vi "read_data_from_fieldpoint.vi"(8 "error in (no error)":errorcluster, 11 "fieldpoint_rw in":refnum<class "fieldpoint_rw.lvclass">) -> (0 "error out":errorcluster, 3 "fieldpoint_rw out":refnum<class "fieldpoint_rw.lvclass">)   [LabVIEW 2015, in "fieldpoint_rw.lvclass"]
uses:
  fieldpoint_rw.lvclass
  fieldpoint_rw.lvclass/fieldpoint_rw.ctl
  <vilib>/FieldPoint/Polymorphic Read.llb/FP Read (Float -IO).vi
panel:
  out "Array":dbl[](array[numeric])
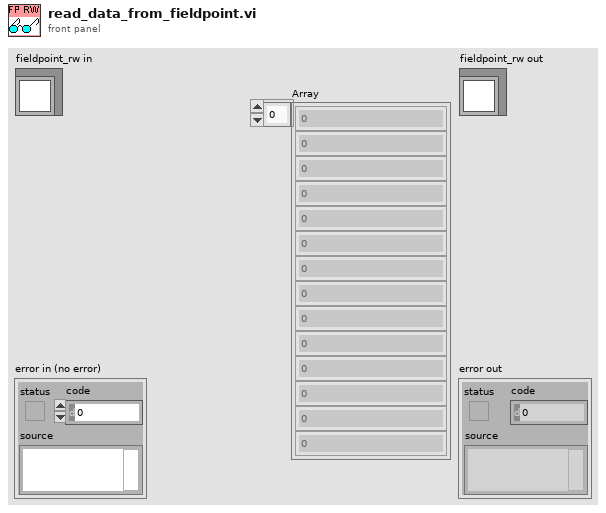
[diagram p1: front panel]
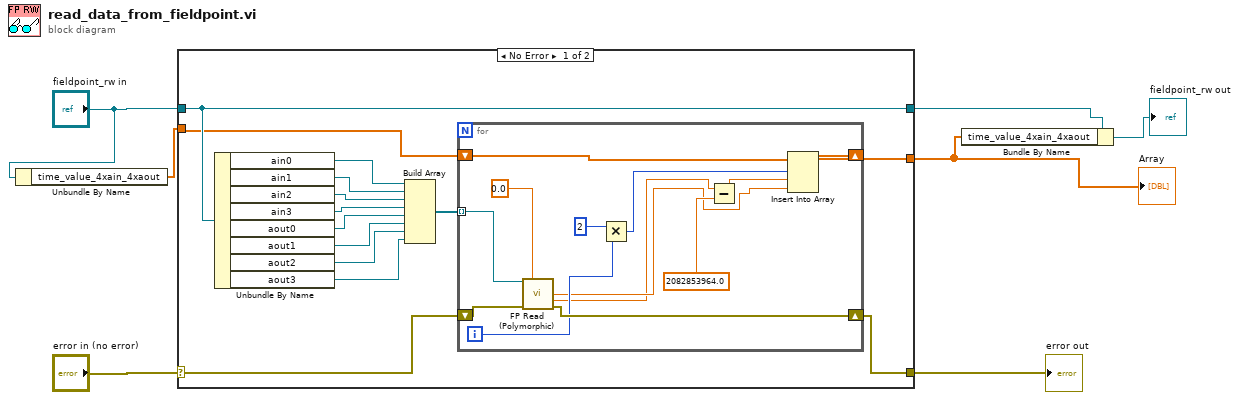
[diagram p0: block diagram]
diagram:
  n1 = Unbundle By Name("fieldpoint_rw in") -> ("time_value_4xain_4xaout"=w4:dbl[])
  n2 = case shown="No Error" "error in (no error)" {
    selector: "error in (no error)" -> [w12 w37]
    tunnel: [w11 w37] -> w6
    tunnel: [w9 w36] -> w3
    tunnel: "fieldpoint_rw in" -> [w9 w36]
    tunnel: [w10 w35] -> w1
    tunnel: w4 -> [w8 w35]
    frame No Error {
      n3 = Unbundle By Name(w9) -> ("ain0"=w21:refnum<k21>, "ain1"=w20:refnum<k21>, "ain2"=w19:refnum<k21>, "ain3"=w18:refnum<k21>, "aout0"=w17:refnum<k21>, "aout1"=w16:refnum<k21>, "aout2"=w15:refnum<k21>, "aout3"=w14:refnum<k21>)
      n4 = Build Array(w21, w20, w19, w18, w17, w16, w15, w14) -> (w13:refnum<k21>[])
      n5 = for {
        tunnel: w13 -> [w33] mode=indexing
        shift-right: [w31] -> w11
        shift-left: w12 -> [w32]
        shift-right: [w26] -> w10
        shift-left: w8 -> [w30]
        i -> [w28]
        n6 = call-poly <vilib>:"FP Read (Polymorphic).vi"("FieldPoint IO Point In"=w33, "Type"=0.0 ("Numeric"), "error in (no error)"=w32) -> ("value"=w24:dbl, "timestamp"=w23:dbl, "error out"=w31:errorcluster)  [unwired: 9 in, 1 out]
        n7 = Multiply(x=2, y=w28) -> (x*y=w27:i32)
        n8 = Subtract(x=w23, y=2082853964.0) -> (x-y=w22:dbl)
        n9 = Insert Into Array(array=w30, index=w27, new element #1=w22, new element #2=w24) -> (w26:dbl[])
      }
    }
    frame Error {
    }
  }
  "error out" <- w6
  "Array" <- w1
  n10 = Bundle By Name(cluster=w3, "time_value_4xain_4xaout"=w1) -> (→"fieldpoint_rw out":refnum<class "fieldpoint_rw.lvclass">)
